vi "Main.vi"() -> ()   [LabVIEW 2015]
doc: "This template is for the Queued Message Handler design pattern.\n\nThe Event Handling Loop generates messages based on user interface actions.\n\nThe Message Handling Loop processes messages generated by the Event Handling Loop, or by other messages. The messages are string values, so new messages can be added easily to the Message Cases case structure in the Message Handling Loop. Each message cluster can also provide an optional value for Message Data, which is a variant that can be converted to whatever message-specific data is required."
uses:
  controls/UI Data.ctl
  support/Message Queue/Enqueue Message (Single).vi
  <vilib>/Utility/error.llb/Error Cluster From Error Code.vi
  <vilib>/ErrorRing/Error Ring.xnode
  support/Message Queue/Message Queue.lvlib
  support/User Events/User Events.lvlib
  <userlib>/cameraLibrary/cameraLibrary.lvlib
panel:
  out "Image":T1(plugin-control)
  out "loopClosed?":bool
  out "ROIUpdated?":bool
  in  "closeLoopButton":bool
  in  "Subframe":dbl(ring) items=["Slow"=0.01, "Medium"=0.005, "Fast"=0.001]
  in  "Full frame":dbl
  out "Y Fiber Position":i32
  out "X Fiber Pos.":i32
  in  "Y Dimension":i16
  in  "X Dimension":i16
  in  "roiButton":bool
  in  "fullFrameButton":bool
  out "Display":string
  in  "abortButton":bool
  in  "subFrameButton":bool
  in  "Exit":bool
  # "Status indicators"
  # "Loop Closed"
  # "ROI Up-to-date"
  # "Timing parameters"
  # "ROI parameters"
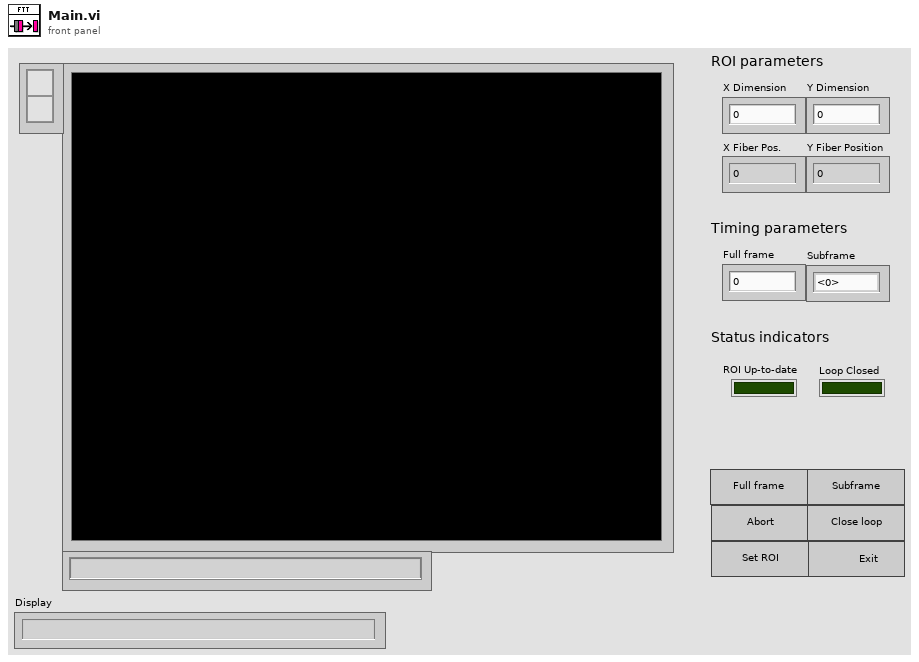
[diagram p1: front panel]
types:
  T1 = typedef "IMAQ Image.ctl" = refnum<image>
  T2 = typedef "Image Type" = u32
  T3 = typedef "UI Data.ctl" = cluster{"full Frame Button Ref":refnum<vi>, "subFrame Button Ref":refnum<vi>, "closed Loop Button Ref":refnum<vi>, "ROI button Ref":refnum<vi>, "abort Button Ref":refnum<vi>, "exit Button Ref":refnum<vi>, "acquiring":bool, " acquiring Ref":refnum<vi>, " ROI Updated Ref":refnum<vi>, "loop Closed Ref":refnum<vi>, "ROI":cluster{"X dimension":i16, "Y dimension":i16, "X binning":i16, "Y binning":i16, "X start":i16, "Y start":i16}, "String <Replace Me>":string, "Data Display Ref":refnum<vi>, "Image Ref":refnum<vi>}
  T4 = typedef "UI Events.ctl" = cluster{"User Event - Stop":refnum<user-event>, "User Event - Abort":refnum<user-event>}
  T5 = typedef "Message Queue.lvlib/All Message Queues.ctl" = cluster{"UI":refnum<queue>, "DataDisplay":refnum<queue>}
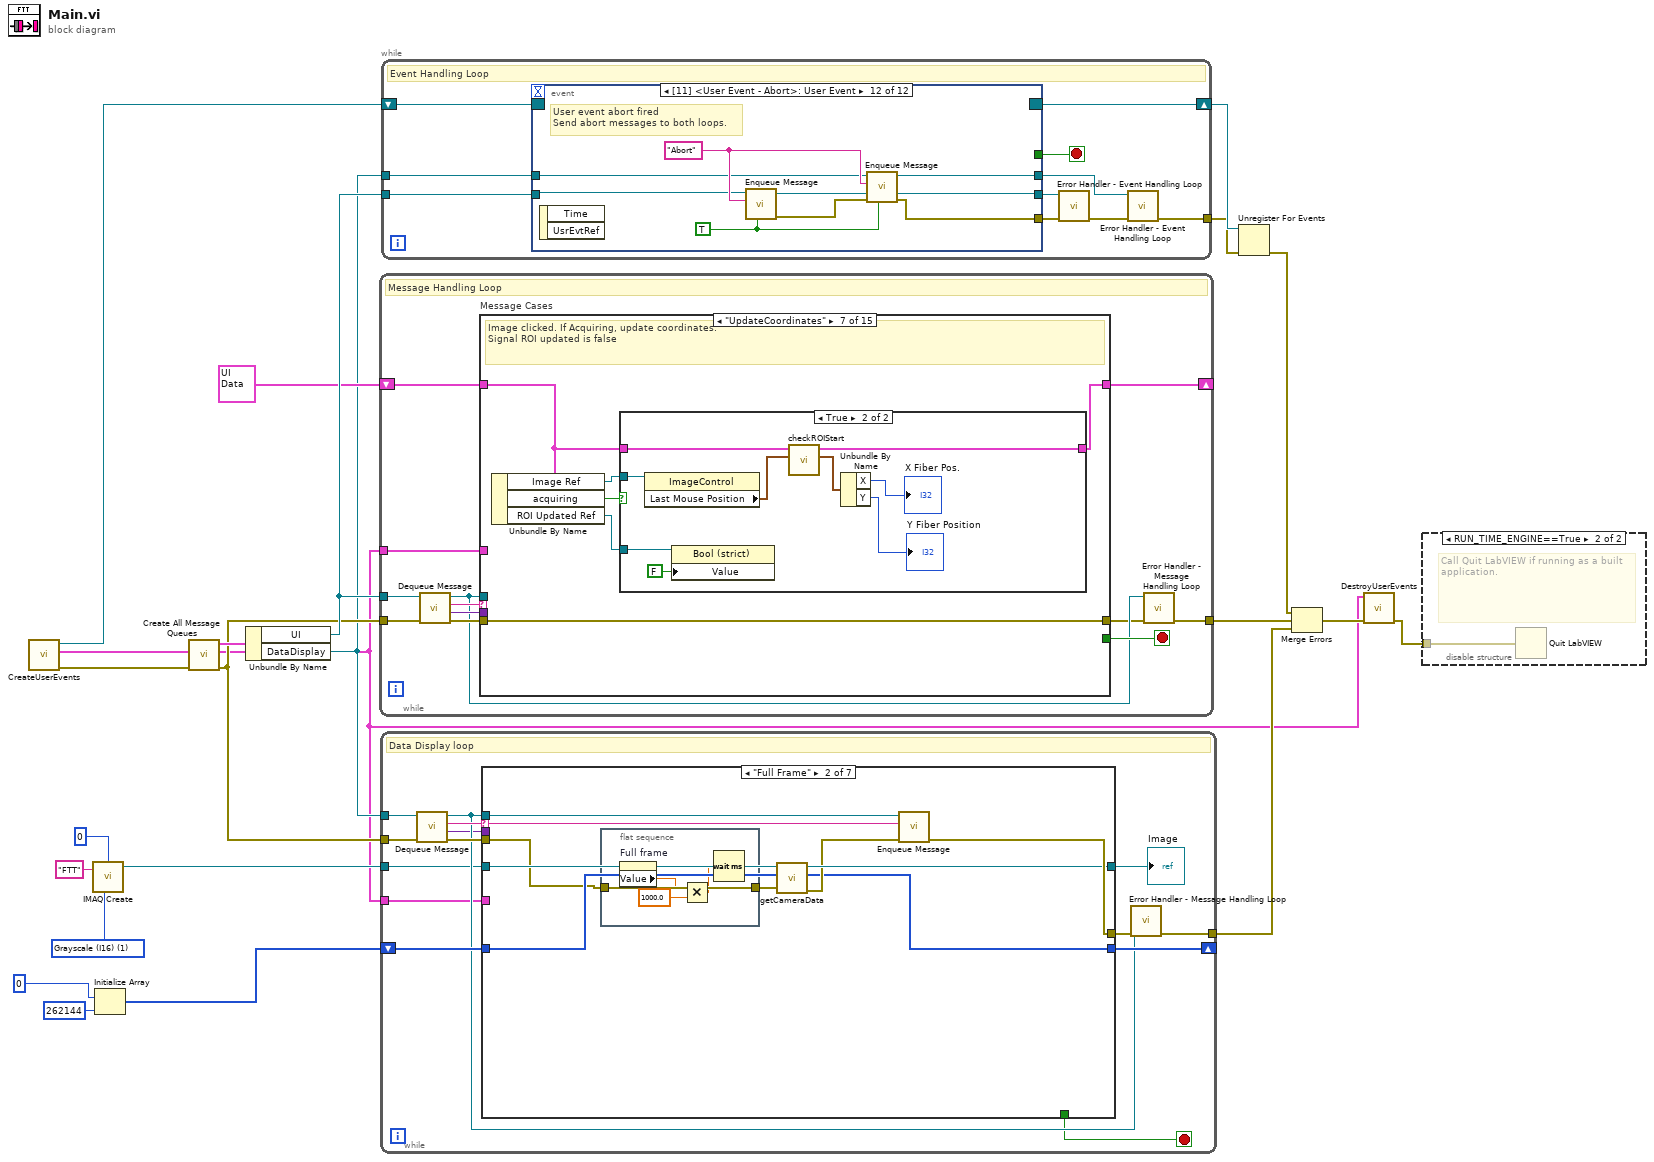
[diagram p0: block diagram]
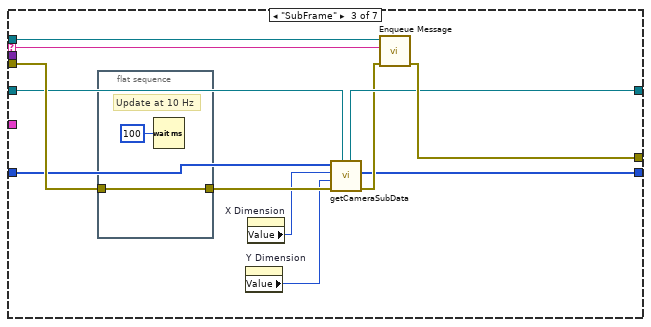
[diagram p3: hidden frame]
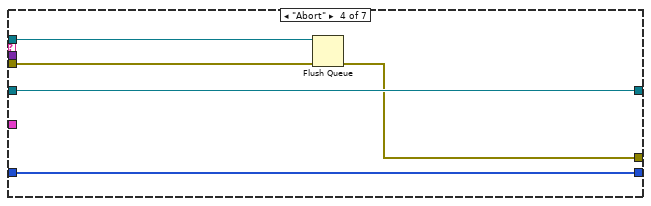
[diagram p4: hidden frame]
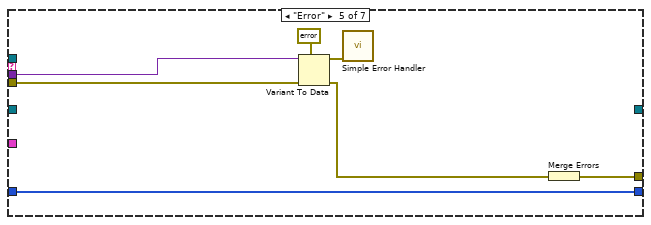
[diagram p5: hidden frame]
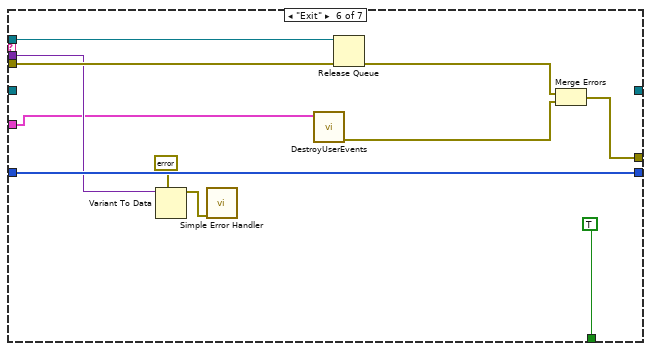
[diagram p6: hidden frame]
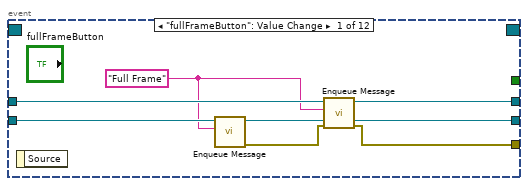
[diagram p9: hidden frame]
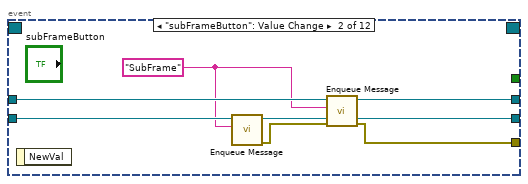
[diagram p10: hidden frame]
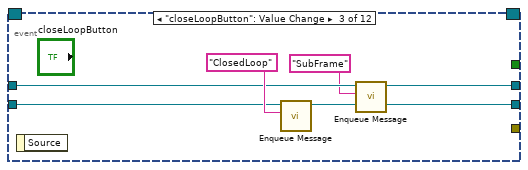
[diagram p11: hidden frame]
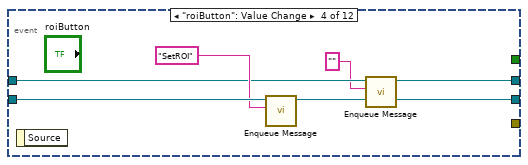
[diagram p12: hidden frame]
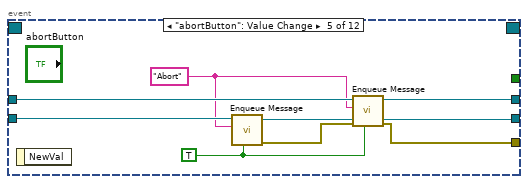
[diagram p13: hidden frame]
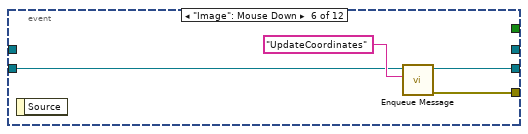
[diagram p14: hidden frame]
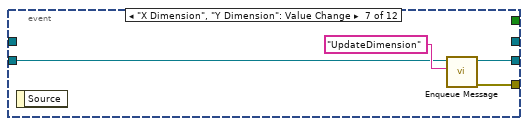
[diagram p15: hidden frame]
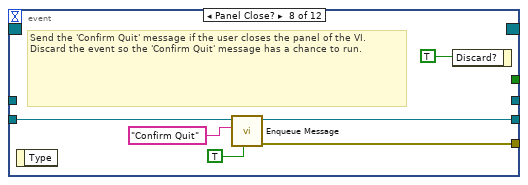
[diagram p16: hidden frame]
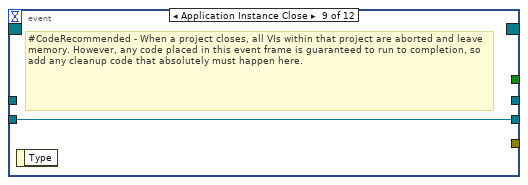
[diagram p17: hidden frame]
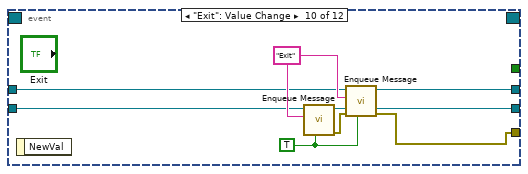
[diagram p18: hidden frame]
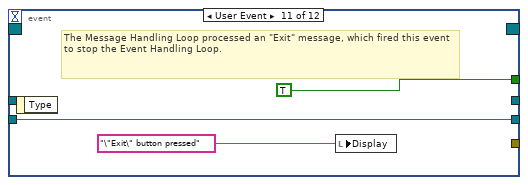
[diagram p19: hidden frame]
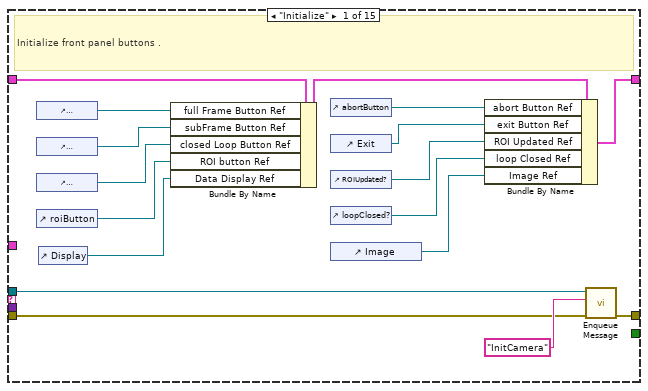
[diagram p20: hidden frame]
diagram:
  w9 = T2 1 items=["Grayscale (U8)", "Grayscale (I16)", "Grayscale (SGL)", "Complex (CSG)", "RGB (U32)", "HSL (U32)", "RGB (U64)", "Grayscale (U16)"] ("Image Type")
  n1 = call "CreateUserEvents.vi"() -> ("error out"=w19:errorcluster, "Event Cluster"=w1:T4, "Event Registration Refnum out"=w15:refnum<event-registration>)  [unwired: 9 in]
  n2 = call "IMAQ Create"("Border Size"=0, "Image Name"="FTT", "Image Type"=w9) -> ("New Image"=w5:T1)  [unwired: 2 in, 1 out]
  n3 = Initialize Array(u32 0, 262144 ("dimension size")) -> (w8:u32[])
  n4 = call "Create All Message Queues.vi"("error in (no error)"=w19) -> ("error out"=w7:errorcluster, "Message Queues out"=w22:T5)  [unwired: 9 in]
  n5 = Unbundle By Name(w22) -> ("UI"=w20:refnum<queue>, "DataDisplay"=w4:refnum<queue>)
  n6 = while {
    tunnel: w20 -> [w29]
    shift-right: [w24] -> _
    shift-left: T3 {"full Frame Button Ref"=refnum, "subFrame Button Ref"=refnum, "closed Loop Button Ref"=refnum, "ROI button Ref"=refnum, "abort Button Ref"=refnum, "exit Button Ref"=refnum, "acquiring"=FALSE, " acquiring Ref"=refnum, " ROI Updated Ref"=refnum, "loop Closed Ref"=refnum, "ROI"={"X dimension"=0, "Y dimension"=0, "X binning"=0, "Y binning"=0, "X start"=0, "Y start"=0}, "String <Replace Me>"="", "Data Display Ref"=refnum, "Image Ref"=refnum} ("Data Cluster") -> [w34]
    tunnel: [w25] -> w21
    tunnel: w7 -> [w26]
    tunnel: w1 -> [w23]
    stop <- w33 stop-if-true
    # "Message Handling Loop"
    n7 = call "Dequeue Message.vi"("error in (no error)"=w26, "Message Queue"=w29) -> ("error out"=w32:errorcluster, "Message Data"=w30:variant, "Message"=w31:string, "dup Message Queue"=w28:refnum<queue>)  [unwired: 6 in]
    n8 = case "Message Cases" shown="\"UpdateCoordinates\"" w31 {
      selector: w31 -> [_ _ w67 _ _ _ _ _ _ _ _ _ _ _ w206]
      tunnel: w28 -> [w48 w62 w70 w86 _ _ _ _ _ _ _ w182 _ w205 _]
      tunnel: w32 -> [w47 w57 w69 w85 w104 w122 w138 w153 w155 w170 w179 w186 w189 w196 _]
      tunnel: [w51 w63 w68 w89 w103 w121 w138 w153 w159 w171 w173 w184 w187 w201 w207] -> w27
      tunnel: w34 -> [w50 w52 w72 w88 w106 w124 w136 w152 w157 w172 w178 w185 w188 w204 w208]
      tunnel: [w41 w60 w66 w90 w105 w123 w135 w151 w158 w172 w178 w185 w188 w204 w208] -> w24
      tunnel: [_ _ _ _ _ _ _ _ _ _ _ _ _ TRUE _] -> w33
      tunnel: w30 -> [_ _ _ _ _ _ _ _ _ w169 w177 _ _ w197 _]
      tunnel: w23 -> [_ _ w65 w84 w102 _ _ _ _ _ _ _ _ w192 _]
      frame "Initialize" {
        # "Initialize front panel buttons ."
        n9 = control-ref of="fullFrameButton"() -> (w46:refnum<vi>)
        n10 = control-ref of="subFrameButton"() -> (w45:refnum<vi>)
        n11 = control-ref of="closeLoopButton"() -> (w44:refnum<vi>)
        n12 = control-ref of="roiButton"() -> (w43:refnum<vi>)
        n13 = control-ref of="Display"() -> (w35:refnum<vi>)
        n14 = Bundle By Name(cluster=w50, "full Frame Button Ref"=w46, "subFrame Button Ref"=w45, "closed Loop Button Ref"=w44, "ROI button Ref"=w43, "Data Display Ref"=w35) -> (w42:T3)
        n15 = control-ref of="abortButton"() -> (w37:refnum<vi>)
        n16 = control-ref of="Exit"() -> (w38:refnum<vi>)
        n17 = control-ref of="ROIUpdated?"() -> (w36:refnum<vi>)
        n18 = control-ref of="loopClosed?"() -> (w39:refnum<vi>)
        n19 = control-ref of="Image"() -> (w40:refnum<vi>)
        n20 = Bundle By Name(cluster=w42, "abort Button Ref"=w37, "exit Button Ref"=w38, "ROI Updated Ref"=w36, "loop Closed Ref"=w39, "Image Ref"=w40) -> (w41:T3)
        n21 = call-poly "Enqueue Message.vi"("error in (no error)"=w47, "Message"="InitCamera", "Message Queue"=w48) -> ("error out"=w51:errorcluster)  [unwired: 7 in, 1 out]
      }
      frame "InitCamera" {
        w54 = 0.00125 items=["Slow"=0.01, "Medium"=0.035, "Fast"=0.00125] ("Subframe")
        w58 = i16 240 ("ROI.X start")
        w59 = i16 1 ("ROI.X binning")
        w55 = i16 32 ("ROI.X dimension")
        n22 = property on="Subframe" class="Ring (strict)"("Value"=w54) -> ()  [unwired: 2 in, 2 out]
        n23 = Bundle By Name(cluster=w52, "ROI.X dimension"=w55, "ROI.Y dimension"=w55, "ROI.X binning"=w59, "ROI.Y binning"=w59, "ROI.X start"=w58, "ROI.Y start"=w58) -> (w60:T3)
        n24 = call <userlib>:"initialize Camera LV.vi"("error in (no error)"=w57) -> ("error out"=w56:errorcluster)  [unwired: 10 in]
        n25 = property on="Full frame" class="DigNum (strict)"("Value"=0.5 ("Full frame")) -> ()  [unwired: 2 in, 2 out]
        n26 = property on="X Dimension" class="DigNum (strict)"("Value"=w55) -> ()  [unwired: 2 in, 2 out]
        n27 = property on="Y Dimension" class="DigNum (strict)"("Value"=w55) -> ()  [unwired: 2 in, 2 out]
        n28 = call-poly "Enqueue Message.vi"("error in (no error)"=w56, "Message Data"="Camera initialized" ("\"Do Something Else\" button pressed"), "Message"="Update Display", "Message Queue"=w62) -> ("error out"=w63:errorcluster)  [unwired: 6 in, 1 out]
      }
      frame "Full Frame" {
        n29 = Unbundle By Name(w72) -> ("acquiring"=w71:bool)
        n30 = case shown="True" w71 {
          tunnel: w72 -> [w77 w82]
          tunnel: [w77 w83] -> w66
          tunnel: w70 -> [_ _]
          tunnel: w69 -> [w74 w78]
          tunnel: [w73 w79] -> w68
          tunnel: w67 -> [_ _]
          tunnel: w65 -> [w76 _]
          frame True {
            # "Currently acquiring.\nFire user abort event."
            n31 = Unbundle By Name(w76) -> ("User Event - Abort"=w75:refnum<user-event>)
            n32 = call "Fire User Event - Abort.vi"("error in (no error)"=w74, "User Event - Abort"=w75) -> ("error out"=w73:errorcluster)  [unwired: 9 in]
          }
          frame False {
            # "Not currently acquiring.\nStart acquisition\nUpdate display parameters"
            n33 = call <userlib>:"acquire Full Frame LV.vi"("error in (no error)"=w78, "expTime"="Full frame") -> ("error out"=w80:errorcluster)  [unwired: 9 in]
            n34 = call "updateGUIDisplayParams.vi"("error in (no error)"=w80, "Data Cluster in"=w82) -> ("error out"=w79:errorcluster, "Data Cluster out"=w83:T3)  [unwired: 8 in]
          }
        }
      }
      frame "SubFrame" {
        # "Acquire a single frame from the camera"
        n35 = Unbundle By Name(w88) -> ("acquiring"=w87:bool)
        n36 = case shown="False" w87 {
          tunnel: w88 -> [w95 w96]
          tunnel: [w95 w99] -> w90
          tunnel: w86 -> [_ _]
          tunnel: w85 -> [w92 w101]
          tunnel: [w91 w97] -> w89
          tunnel: w84 -> [w94 _]
          frame True {
            # "Currently acquiring.\nFire user abort event.\nAborts current acquisition and stops data display loop"
            n37 = Unbundle By Name(w94) -> ("User Event - Abort"=w93:refnum<user-event>)
            n38 = call "Fire User Event - Abort.vi"("error in (no error)"=w92, "User Event - Abort"=w93) -> ("error out"=w91:errorcluster)  [unwired: 9 in]
          }
          frame False {
            n39 = call <userlib>:"acquire Sub Frame LV.vi"("error in (no error)"=w101, "expTime"="Subframe") -> ("error out"=w98:errorcluster)  [unwired: 9 in]
            n40 = call "updateGUIDisplayParams.vi"("error in (no error)"=w98, "Data Cluster in"=w96) -> ("error out"=w97:errorcluster, "Data Cluster out"=w99:T3)  [unwired: 8 in]
          }
        }
      }
      frame "ClosedLoop" {
        # "Handle closed loop button press. Start process FTT loop."
        n41 = Unbundle By Name(w106) -> ("acquiring"=w107:bool)
        n42 = case shown="True" w107 {
          tunnel: w106 -> [w112 w120]
          tunnel: [w109 w120] -> w105
          tunnel: w104 -> [w115 w117]
          tunnel: [w110 w116] -> w103
          tunnel: w102 -> [_ w119]
          frame False {
            # "Not acquiring, start closed\nloop acquisition"
            n43 = property on="Subframe" class="Ring (strict)"(error in=w115) -> (error out=w114:errorcluster, "Value"=w113:dbl)  [unwired: 1 in, 1 out]
            n44 = call <userlib>:"acquire Closed Loop LV.vi"("error in (no error)"=w114, "expTime"=w113) -> ("error out"=w111:errorcluster)  [unwired: 9 in]
            n45 = call "updateGUIDisplayParams.vi"("error in (no error)"=w111, "Data Cluster in"=w112) -> ("error out"=w110:errorcluster, "Data Cluster out"=w109:T3)  [unwired: 8 in]
            "loopClosed?" <- TRUE ("loopClosed?")
          }
          frame True {
            # "Currently acquiring.\nFire user abort event.\nAborts current acquisition and stops data display loop"
            n46 = Unbundle By Name(w119) -> ("User Event - Abort"=w118:refnum<user-event>)
            n47 = call "Fire User Event - Abort.vi"("error in (no error)"=w117, "User Event - Abort"=w118) -> ("error out"=w116:errorcluster)  [unwired: 9 in]
          }
        }
      }
      frame "SetROI" {
        # "Program camera with ROI values."
        n48 = Unbundle By Name(w124) -> ("acquiring"=w125:bool)
        n49 = case shown="True" w125 {
          tunnel: w124 -> [w127 w132]
          tunnel: [w127 w131] -> w123
          tunnel: w122 -> [w126 w130]
          tunnel: [w126 w129] -> w121
          frame True {
            # "Acquiring, do nothing\nShould be fixed with button masking"
          }
          frame False {
            # "Not acquiring, set ROI"
            n50 = call "setROI.vi"("error in (no error)"=w130, "FTTclusterIn"=w132) -> ("error out"=w129:errorcluster, "FTTclusterOut"=w131:T3)  [unwired: 8 in]
            "ROIUpdated?" <- TRUE ("ROIUpdated?")
          }
        }
      }
      frame "UpdateCoordinates" {
        # "Image clicked. If Acquiring, update coordinates.\nSignal ROI updated is false"
        n51 = Unbundle By Name(w136) -> ("Image Ref"=w133:refnum<vi>, "acquiring"=w137:bool, "ROI Updated Ref"=w134:refnum<vi>)
        n52 = case shown="True" w137 {
          tunnel: w136 -> [w139 w147]
          tunnel: [w139 w146] -> w135
          tunnel: w134 -> [_ w142]
          tunnel: w133 -> [_ w140]
          frame False {
          }
          frame True {
            n53 = property class="ImageControl"(reference=w140) -> ("Last Mouse Position"=w148:cluster{"X":i32, "Y":i32})  [unwired: 1 in, 2 out]
            n54 = property class="Bool (strict)"(reference=w142, "Value"=FALSE) -> ()  [unwired: 1 in, 2 out]
            n55 = call "checkROIStart.vi"("lastClickPosition"=w148, "FTTDataClusterIn"=w147) -> ("coords"=w145:cluster{"X":i32, "Y":i32}, "FTTDataClusterOut"=w146:T3)  [unwired: 8 in]
            n56 = Unbundle By Name(w145) -> ("X"=→"X Fiber Pos.":i32, "Y"=→"Y Fiber Position":i32)
          }
        }
      }
      frame "UpdateDimension" {
        n57 = Bundle By Name(cluster=w152, "ROI.X dimension"="X Dimension", "ROI.Y dimension"="Y Dimension") -> (w151:T3)
      }
      frame "Abort" {
        # "Abort camera acquistion and update GUI."
        n58 = Unbundle By Name(w157) -> ("acquiring"=w156:bool)
        n59 = call <userlib>:"abort Acquisition LV.vi"("error in (no error)"=w155) -> ("error out"=w154:errorcluster)  [unwired: 10 in]
        n60 = case shown="True" w156 {
          tunnel: w154 -> [w161 w165]
          tunnel: [w161 w164] -> w159
          tunnel: [w160 w162] -> w158
          tunnel: w157 -> [w160 w163]
          frame False {
          }
          frame True {
            n61 = call "updateGUIDisplayParams.vi"("error in (no error)"=w165, "Data Cluster in"=w163) -> ("error out"=w164:errorcluster, "Data Cluster out"=w162:T3)  [unwired: 8 in]
          }
        }
      }
      frame "Update Display" {
        # "Update Display - Convert the message data to a string to display in the Data Display indicator."
        n62 = Variant To Data(error in=w170, type="", Variant=w169) -> (data=→"Display":string, error out=w167:errorcluster)
        n63 = Merge Errors(w167) -> (w171:errorcluster)
      }
      frame "Error" {
        # "#CodeRecommended - If you ever change the name of this \"Error\" message, you'll need to update the name in the Check Loop Error.vi as well."
        # "#CodeRecommended - Consider creating a system for logging errors in some way. These errors are for notification purposes only. Handling of specific errors should be performed in the message frames that generated the error."
        # "Error - Display an error dialog. This message is sent by the \"Error Handler\" VIs at the end of other loops in this application."
        n64 = Variant To Data(error in=w179, type=errorcluster {"status"=FALSE, "code"=0, "source"=""} ("error constant"), Variant=w177) -> (data=w175:errorcluster, error out=w174:errorcluster)
        n65 = call <vilib>:"Simple Error Handler.vi"("error in (no error)"=w175) -> ()  [unwired: 4 in, 5 out]
        n66 = Merge Errors(w174) -> (w173:errorcluster)
      }
      frame "Confirm Quit" {
        # "#CodeNeeded - If you want to provide an \"Are you sure\" dialog (or some other notification) before the application exits, place that code here. This message is typically sent from a Panel Close? event."
        # "Confirm Quit - Message that can confirm whether or not the user wants to exit the application."
        n67 = call-poly "Enqueue Message.vi"("Priority Message? (F)"=TRUE, "error in (no error)"=w186, "Message"="Exit", "Message Queue"=w182) -> ("error out"=w183:errorcluster)  [unwired: 6 in, 1 out]
        n68 = Merge Errors(w183) -> (w184:errorcluster)
      }
      frame "---Copy This Frame---" {
        # "Duplicate this frame when creating new messages.  Change this comment in the duplicated frame to describe this message."
        n69 = Merge Errors(w189) -> (w187:errorcluster)
      }
      frame "Exit" {
        # "Stop the VI"
        # "#CodeNeeded - Add any required cleanup code here. Note that if 'Exit' was called as a result of an error, an error dialog will be displayed. Add any custom error handling for an 'Exit' condition here as well."
        # "Exit - Exit the application."
        n70 = Unbundle By Name(w192) -> ("User Event - Stop"=w191:refnum<user-event>, "User Event - Abort"=w190:refnum<user-event>)
        n71 = Variant To Data(type=errorcluster {"status"=FALSE, "code"=0, "source"=""} ("error constant"), Variant=w197) -> (data=w198:errorcluster)  [unwired: 1 in, 1 out]
        n72 = call <vilib>:"Simple Error Handler.vi"("error in (no error)"=w198) -> ()  [unwired: 4 in, 5 out]
        n73 = call <userlib>:"abort Acquisition LV.vi"("error in (no error)"=w196) -> ("error out"=w195:errorcluster)  [unwired: 10 in]
        n74 = call <userlib>:"shutdown Camera LV.vi"("error in (no error)"=w195) -> ("error out"=w194:errorcluster)  [unwired: 10 in]
        n75 = call "Destroy User Event -Abort.vi"("User Event - Abort"=w190) -> ("error out"=w193:errorcluster)  [unwired: 10 in]
        n76 = call "Fire User Event - Stop.vi"("error in (no error)"=w193, "User Event - Stop"=w191) -> ("error out"=w200:errorcluster)  [unwired: 9 in]
        n77 = Release Queue(queue=w205, error in (no error)=w194) -> (error out=w202:errorcluster)  [unwired: 1 in, 2 out]
        n78 = Merge Errors(w200, w202) -> (w201:errorcluster)
      }
      frame Default {
        # "'Default' case only runs if there is a message that isn't defined in any of the other cases.  Output a programming error."
        n79 = xnode "Error Ring"("parameter 0"=w206) -> ("error out"=w207:errorcluster)
      }
    }
    n80 = call "Error Handler - Message Handling Loop.vi"("error in (no error)"=w27, "Message Queue"=w28) -> ("dup error in"=w25:errorcluster)  [unwired: 8 in, 1 out]
  }
  n81 = while {
    tunnel: w4 -> [w228]
    tunnel: w7 -> [w227]
    tunnel: [w225] -> w6
    shift-right: [w222] -> _
    shift-left: w8 -> [w229]
    tunnel: w5 -> [w219]
    tunnel: w1 -> [w216]
    stop <- w220 stop-if-true
    # "Data Display loop"
    n82 = call "Dequeue Message.vi"("error in (no error)"=w227, "Message Queue"=w228) -> ("error out"=w223:errorcluster, "Message Data"=w218:variant, "Message"=w226:string, "dup Message Queue"=w221:refnum<queue>)  [unwired: 6 in]
    n83 = case shown="\"Full Frame\"" w226 {
      selector: w226 -> [_ w241 w257 _ _ _ _]
      tunnel: w229 -> [w232 w236 w253 w263 w268 w278 w285]
      tunnel: w221 -> [_ w242 w258 w265 _ w283 _]
      tunnel: [w231 w240 w256 w261 w266 w281 w286] -> w224
      tunnel: w223 -> [w231 w234 w255 w264 w270 w282 w286]
      tunnel: [w230 w238 w251 w262 _ _ w284] -> w217
      tunnel: [w232 w235 w249 w263 w268 w278 w285] -> w222
      tunnel: [_ _ _ _ _ TRUE _] -> w220
      tunnel: w219 -> [w230 w239 w252 w262 _ _ w284]
      tunnel: w218 -> [_ _ _ _ w269 w276 _]
      tunnel: w216 -> [_ _ _ _ _ w273 _]
      frame "Initialize" {
      }
      frame "Full Frame" {
        n84 = flat-sequence {
          tunnel: w234 -> [w246]
          tunnel: [w246] -> w233
          frame #0 {
            n85 = property on="Full frame" class="DigNum (strict)"() -> ("Value"=w244:dbl)  [unwired: 2 in, 2 out]
            n86 = Multiply(x=w244, y=1000.0) -> (x*y=w245:dbl)
            n87 = Wait (ms)(milliseconds to wait=w245) -> ()  [unwired: 1 out]
          }
        }
        n88 = call "getCameraData.vi"("error in (no error)"=w233, "Array"=w236, "Refnum in"=w239) -> ("error out"=w237:errorcluster, "arrayOut"=w235:u32[], "Refnum out"=w238:T1)  [unwired: 6 in]
        n89 = call-poly "Enqueue Message.vi"("error in (no error)"=w237, "Message"=w241, "Message Queue"=w242) -> ("error out"=w240:errorcluster)  [unwired: 7 in, 1 out]
      }
      frame "SubFrame" {
        n90 = flat-sequence {
          tunnel: w255 -> [w259]
          tunnel: [w259] -> w254
          frame #0 {
            # "Update at 10 Hz"
            n91 = Wait (ms)(milliseconds to wait=u32 100) -> ()  [unwired: 1 out]
          }
        }
        n92 = property on="Y Dimension" class="DigNum (strict)"() -> ("Value"=w248:i16)  [unwired: 2 in, 2 out]
        n93 = property on="X Dimension" class="DigNum (strict)"() -> ("Value"=w247:i16)  [unwired: 2 in, 2 out]
        n94 = call "getCameraSubData.vi"("Refnum in"=w252, "error in (no error)"=w254, "VDim"=w248, "HDim"=w247, "arrayIn"=w253) -> ("error out"=w250:errorcluster, "arrayOut"=w249:u32[], "Refnum out"=w251:T1)  [unwired: 4 in]
        n95 = call-poly "Enqueue Message.vi"("error in (no error)"=w250, "Message"=w257, "Message Queue"=w258) -> ("error out"=w256:errorcluster)  [unwired: 7 in, 1 out]
      }
      frame "Abort" {
        n96 = Flush Queue(queue=w265, error in (no error)=w264) -> (error out=w261:errorcluster)  [unwired: 2 out]
      }
      frame "Error" {
        n97 = Variant To Data(error in=w270, type=errorcluster {"status"=FALSE, "code"=0, "source"=""} ("error constant"), Variant=w269) -> (data=w271:errorcluster, error out=w267:errorcluster)
        n98 = call <vilib>:"Simple Error Handler.vi"("error in (no error)"=w271) -> ()  [unwired: 4 in, 5 out]
        n99 = Merge Errors(w267) -> (w266:errorcluster)
      }
      frame "Exit" {
        n100 = Variant To Data(type=errorcluster {"status"=FALSE, "code"=0, "source"=""} ("error constant"), Variant=w276) -> (data=w277:errorcluster)  [unwired: 1 in, 1 out]
        n101 = call <vilib>:"Simple Error Handler.vi"("error in (no error)"=w277) -> ()  [unwired: 4 in, 5 out]
        n102 = call "DestroyUserEvents.vi"("Event Cluster"=w273) -> ("error out"=w280:errorcluster)  [unwired: 10 in]
        n103 = Release Queue(queue=w283, error in (no error)=w282) -> (error out=w274:errorcluster)  [unwired: 1 in, 2 out]
        n104 = Merge Errors(w274, w280) -> (w281:errorcluster)
      }
      frame Default {
      }
    }
    "Image" <- w217
    n105 = call "Error Handler - Message Handling Loop.vi"("error in (no error)"=w224, "Message Queue"=w221) -> ("dup error in"=w225:errorcluster)  [unwired: 8 in, 1 out]
  }
  n106 = while {
    tunnel: w20 -> [w296]
    shift-right: [w294] -> w18
    shift-left: w15 -> [w295]
    tunnel: [w289] -> w16
    tunnel: w4 -> [w291]
    stop <- w293 stop-if-true
    # "Event Handling Loop"
    n107 = event shown="[11] <User Event - Abort>: User Event" {
      selector: w295 -> [_ _ _ _ _ _ _ _ _ _ _ _]
      dyn-events: [_ _ _ _ _ _ _ _ _ _ _ _] -> w294
      timeout: _ -> [_ _ _ _ _ _ _ _ _ _ _ _]
      tunnel: [_ _ _ _ _ _ _ _ _ _ TRUE ("Discard?") _] -> w293
      tunnel: w296 -> [w303 w310 w315 w322 w330 w333 w337 w343 w345 w349 w356 w359]
      tunnel: [w299 w306 _ _ w325 w331 w335 w342 _ w346 _ w357] -> w287
      tunnel: [w302 w309 w314 w321 w329 w332 w336 w341 w345 w353 w356 w360] -> w292
      tunnel: w291 -> [w301 w308 w312 w319 w328 _ _ _ _ w348 _ w358]
      tunnel: [w298 w304 w313 w318 w326 _ _ _ _ w350 _ w361] -> w288
      event "fullFrameButton": Value Change {
        w297 = "Full Frame" ("Message")
        n108 = event-data() -> ()  [unwired: 1 in, 1 out]
        n109 = call-poly "Enqueue Message.vi"("Message"=w297, "Message Queue"=w303) -> ("error out"=w300:errorcluster, "dup Message Queue"=w302:refnum<queue>)  [unwired: 8 in]
        n110 = call-poly "Enqueue Message.vi"("error in (no error)"=w300, "Message"=w297, "Message Queue"=w301) -> ("error out"=w299:errorcluster, "dup Message Queue"=w298:refnum<queue>)  [unwired: 7 in]
      }
      event "subFrameButton": Value Change {
        w305 = "SubFrame" ("Message")
        n111 = event-data() -> ()  [unwired: 1 in, 1 out]
        n112 = call-poly "Enqueue Message.vi"("Message"=w305, "Message Queue"=w310) -> ("error out"=w307:errorcluster, "dup Message Queue"=w309:refnum<queue>)  [unwired: 8 in]
        n113 = call-poly "Enqueue Message.vi"("error in (no error)"=w307, "Message"=w305, "Message Queue"=w308) -> ("error out"=w306:errorcluster, "dup Message Queue"=w304:refnum<queue>)  [unwired: 7 in]
      }
      event "closeLoopButton": Value Change {
        n114 = event-data() -> ()  [unwired: 1 in, 1 out]
        n115 = call-poly "Enqueue Message.vi"("Message"="ClosedLoop", "Message Queue"=w315) -> ("dup Message Queue"=w314:refnum<queue>)  [unwired: 8 in, 1 out]
        n116 = call-poly "Enqueue Message.vi"("Message"="SubFrame", "Message Queue"=w312) -> ("dup Message Queue"=w313:refnum<queue>)  [unwired: 8 in, 1 out]
      }
      event "roiButton": Value Change {
        n117 = event-data() -> ()  [unwired: 1 in, 1 out]
        n118 = call-poly "Enqueue Message.vi"("Message"="SetROI", "Message Queue"=w322) -> ("dup Message Queue"=w321:refnum<queue>)  [unwired: 8 in, 1 out]
        n119 = call-poly "Enqueue Message.vi"("Message"="", "Message Queue"=w319) -> ("dup Message Queue"=w318:refnum<queue>)  [unwired: 8 in, 1 out]
      }
      event "abortButton": Value Change {
        w323 = TRUE ("Priority Message? (F)")
        w324 = "Abort" ("Message")
        n120 = event-data() -> ()  [unwired: 1 in, 1 out]
        n121 = call-poly "Enqueue Message.vi"("Priority Message? (F)"=w323, "Message"=w324, "Message Queue"=w330) -> ("error out"=w327:errorcluster, "dup Message Queue"=w329:refnum<queue>)  [unwired: 7 in]
        n122 = call-poly "Enqueue Message.vi"("Priority Message? (F)"=w323, "error in (no error)"=w327, "Message"=w324, "Message Queue"=w328) -> ("error out"=w325:errorcluster, "dup Message Queue"=w326:refnum<queue>)  [unwired: 6 in]
      }
      event "Image": Mouse Down {
        n123 = event-data() -> ()  [unwired: 1 in, 1 out]
        n124 = call-poly "Enqueue Message.vi"("Message"="UpdateCoordinates", "Message Queue"=w333) -> ("error out"=w331:errorcluster, "dup Message Queue"=w332:refnum<queue>)  [unwired: 8 in]
      }
      event "X Dimension", "Y Dimension": Value Change {
        n125 = event-data() -> ()  [unwired: 1 in, 1 out]
        n126 = call-poly "Enqueue Message.vi"("Message"="UpdateDimension", "Message Queue"=w337) -> ("error out"=w335:errorcluster, "dup Message Queue"=w336:refnum<queue>)  [unwired: 8 in]
      }
      event Panel Close? {
        # "Send the 'Confirm Quit' message if the user closes the panel of the VI. Discard the event so the 'Confirm Quit' message has a chance to run."
        n127 = event-data() -> ()  [unwired: 1 in, 1 out]
        n128 = call-poly "Enqueue Message.vi"("Priority Message? (F)"=TRUE, "Message"="Confirm Quit", "Message Queue"=w343) -> ("error out"=w342:errorcluster, "dup Message Queue"=w341:refnum<queue>)  [unwired: 7 in]
        n129 = event-data("Discard?"=TRUE) -> ()  [unwired: 1 in, 1 out]
      }
      event Application Instance Close {
        # "#CodeRecommended - When a project closes, all VIs within that project are aborted and leave memory. However, any code placed in this event frame is guaranteed to run to completion, so add any cleanup code that absolutely must happen here."
        n130 = event-data() -> ()  [unwired: 1 in, 1 out]
      }
      event "Exit": Value Change {
        w347 = TRUE ("Priority Message? (F)")
        w351 = "Exit" ("Message")
        n131 = event-data() -> ()  [unwired: 1 in, 1 out]
        n132 = call-poly "Enqueue Message.vi"("Priority Message? (F)"=w347, "Message"=w351, "Message Queue"=w349) -> ("error out"=w352:errorcluster, "dup Message Queue"=w353:refnum<queue>)  [unwired: 7 in]
        n133 = call-poly "Enqueue Message.vi"("Priority Message? (F)"=w347, "error in (no error)"=w352, "Message"=w351, "Message Queue"=w348) -> ("error out"=w346:errorcluster, "dup Message Queue"=w350:refnum<queue>)  [unwired: 6 in]
      }
      event User Event {
        # "The Message Handling Loop processed an \"Exit\" message, which fired this event to stop the Event Handling Loop."
        n134 = event-data() -> ()  [unwired: 1 in, 1 out]
        n135 = local write "Display"("\"Exit\" button pressed" ("VI Stopped")) -> ()
      }
      event User Event {
        w362 = TRUE ("Priority Message? (F)")
        w363 = "Abort" ("Message")
        # "User event abort fired\nSend abort messages to both loops."
        n136 = event-data() -> ()  [unwired: 1 in, 2 out]
        n137 = call-poly "Enqueue Message.vi"("Priority Message? (F)"=w362, "Message"=w363, "Message Queue"=w359) -> ("error out"=w364:errorcluster, "dup Message Queue"=w360:refnum<queue>)  [unwired: 7 in]
        n138 = call-poly "Enqueue Message.vi"("Priority Message? (F)"=w362, "error in (no error)"=w364, "Message"=w363, "Message Queue"=w358) -> ("error out"=w357:errorcluster, "dup Message Queue"=w361:refnum<queue>)  [unwired: 6 in]
      }
    }
    n139 = call "Error Handler - Event Handling Loop.vi"("error in (no error)"=w287, "Message Queue"=w292) -> ("dup error in"=w290:errorcluster)  [unwired: 8 in, 1 out]
    n140 = call "Error Handler - Event Handling Loop.vi"("error in (no error)"=w290, "Message Queue"=w288) -> ("dup error in"=w289:errorcluster)  [unwired: 8 in, 1 out]
  }
  n141 = Unregister For Events(event registration refnum=w18, error in=w16) -> (error out=w14:errorcluster)
  n142 = Merge Errors(w14, w21, w6) -> (w3:errorcluster)
  n143 = call "DestroyUserEvents.vi"("error in (no error)"=w3, "Event Cluster"=w1) -> ("error out"=w2:errorcluster)  [unwired: 9 in]
  n144 = disable-structure shown="RUN_TIME_ENGINE==True" {
    disable-tunnel: w2 -> [_ w365]
    frame condition #0 (active) {
    }
    frame condition #1 {
      # "Call Quit LabVIEW if running as a built application."
      n145 = Quit LabVIEW(quit? (T)=w365) -> ()
    }
  }
